vi "GetWindowSizeInPixels.vi"(8 "No Error":errorcluster, 11 "Window [SDL_Window *]":i64) -> (0 "Error Out":errorcluster, 2 "h":i32, 3 "w":i32)   [LabVIEW 2024, in "SDL3.lvlib" / "Video.lvlib"]
doc: "<B>Summary</B>\nGet the size of a window's client area, in pixels."
uses:
  Video.lvlib
  Lib/SDL3-32.dll
  Error/Error.lvlib
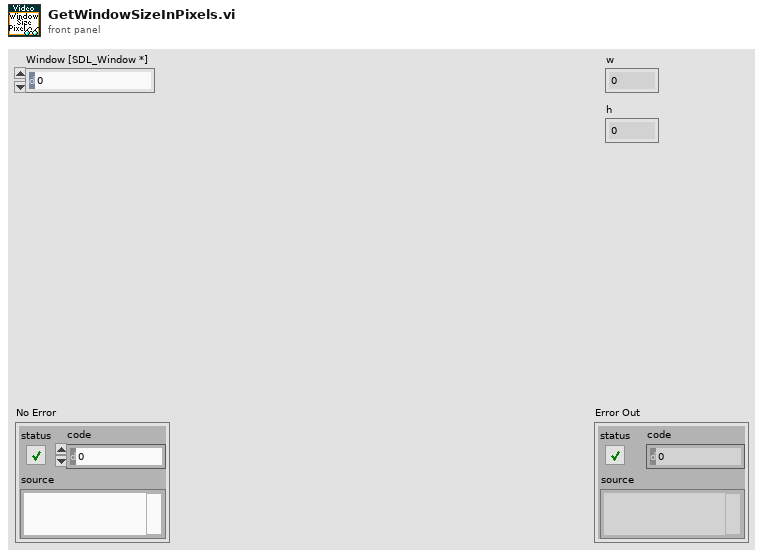
[diagram p1: front panel]
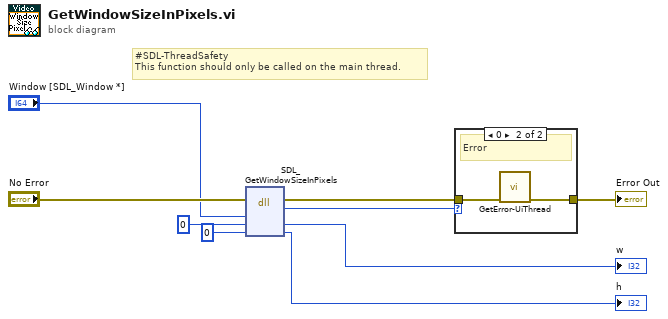
[diagram p0: block diagram]
diagram:
  # "#SDL-ThreadSafety\nThis function should only be called on the main thread."
  n1 = dll-call lib="C:/Users/Thomas/Documents/Projects/LV-SDL3/Lib/SDL3-*.*" fn="SDL_GetWindowSizeInPixels"(error in="No Error", "window"="Window [SDL_Window *]", "w"=0 ("W"), "h"=0 ("H")) -> (error out=w4:errorcluster, "return type"=w3:i32, "w"=→"w":i32, "h"=→"h":i32)  [unwired: 3 in, 1 out]
  n2 = case shown="0" w3 {
    tunnel: w4 -> [w10 w12]
    tunnel: [w10 w11] -> w8
    frame Default {
      # "Ok"
    }
    frame 0 {
      # "Error"
      n3 = call "GetError-UiThread.vi"("No Error"=w12) -> ("error out"=w11:errorcluster)  [unwired: 10 in]
    }
  }
  "Error Out" <- w8
